vi "Sense.vi"(0 "Enum":enum16{"Running", "Impact", "Spinning", "Clear"}(ring)) -> ()   [LabVIEW 2010]
uses:
  Streaming Data.ctl
  Main Global.vi
panel:
  out "Streaming Data":T1
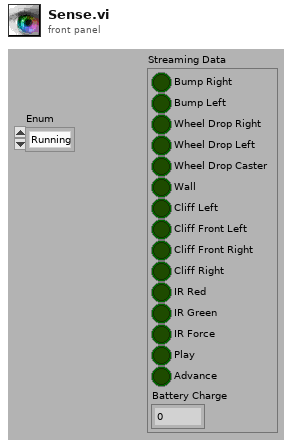
[diagram p1: front panel]
types:
  T1 = typedef "Streaming Data.ctl" = cluster{"Bump Right":bool, "Bump Left":bool, "Wheel Drop Right":bool, "Wheel Drop Left":bool, "Wheel Drop Caster":bool, "Wall":bool, "Cliff Left":bool, "Cliff Front Left":bool, "Cliff Front Right":bool, "Cliff Right":bool, "IR Red":bool, "IR Green":bool, "IR Force":bool, "Play":bool, "Advance":bool, "Battery Charge":i16}
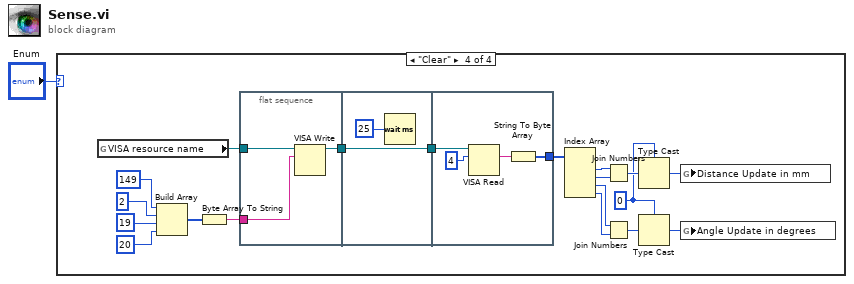
[diagram p0: block diagram]
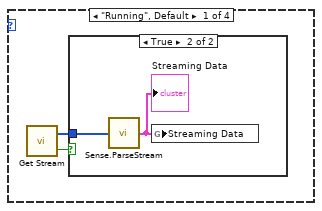
[diagram p2: hidden frame]
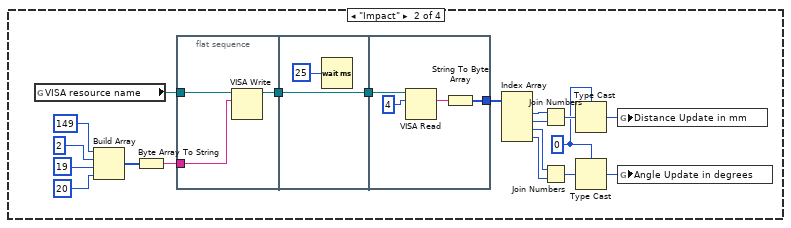
[diagram p4: hidden frame]
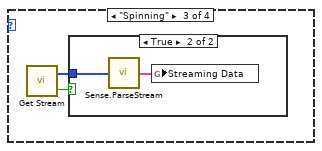
[diagram p5: hidden frame]
diagram:
  n1 = case shown="\"Clear\"" "Enum" {
    frame "Running", Default {
      n2 = call "Get Stream.vi"() -> ("Good Data"=w2:bool, "UART Stream 2"=w3:u8[])  [unwired: 2 in]
      n3 = case shown="True" w2 {
        tunnel: w3 -> [_ w4]
        frame False {
        }
        frame True {
          n4 = call "Sense.ParseStream.vi"("UART Stream"=w4) -> ("Streaming Data"=w5:T1)
          "Streaming Data" <- w5
          n5 = global write "Main Global.vi" "Streaming Data"(w5) -> ()
        }
      }
    }
    frame "Impact" {
      w8 = i16 0
      n6 = global read "Main Global.vi" "VISA resource name"() -> (w24:refnum<visa-resource-name>)
      n7 = Build Array(u8 149, u8 2 ("element"), u8 19, u8 20) -> (w22:u8[])
      n8 = Byte Array To String(unsigned byte array=w22) -> (string=w21:string)
      n9 = flat-sequence {
        tunnel: w24 -> [w27]
        tunnel: w21 -> [w26]
        tunnel: [w25] -> w19
        tunnel: [w28] -> w20
        tunnel: w19 -> [w28]
        tunnel: w20 -> [w33]
        tunnel: [w30] -> w18
        frame #0 {
          n10 = VISA Write(VISA resource name=w27, write buffer=w26) -> (VISA resource name out=w25:refnum<visa-resource-name>)  [unwired: 1 in, 2 out]
        }
        frame #1 {
          n11 = Wait (ms)(milliseconds to wait=u32 25) -> ()  [unwired: 1 out]
        }
        frame #2 {
          n12 = VISA Read(VISA resource name=w33, byte count=u32 4) -> (read buffer=w31:string)  [unwired: 1 in, 3 out]
          n13 = String To Byte Array(string=w31) -> (unsigned byte array=w30:u8[])
        }
      }
      n14 = Index Array(array=w18) -> (element #1=w17:u8, element #2=w16:u8, element #3=w11:u8, element #4=w10:u8)  [unwired: 4 in]
      n15 = Join Numbers(hi=w17, lo=w16) -> ((hi.lo)=w15:u16)
      n16 = Join Numbers(hi=w11, lo=w10) -> ((hi.lo)=w7:u16)
      n17 = Type Cast(type=w8, x=w15) -> (*(type *) &x=w9:i16)
      n18 = Type Cast(type=w8, x=w7) -> (*(type *) &x=w6:i16)
      n19 = global write "Main Global.vi" "Distance Update in mm"(w9) -> ()
      n20 = global write "Main Global.vi" "Angle Update in degrees"(w6) -> ()
    }
    frame "Spinning" {
      n21 = call "Get Stream.vi"() -> ("Good Data"=w35:bool, "UART Stream 2"=w34:u8[])  [unwired: 2 in]
      n22 = case shown="True" w35 {
        tunnel: w34 -> [_ w36]
        frame False {
        }
        frame True {
          n23 = call "Sense.ParseStream.vi"("UART Stream"=w36) -> ("Streaming Data"=w37:T1)
          n24 = global write "Main Global.vi" "Streaming Data"(w37) -> ()
        }
      }
    }
    frame "Clear" {
      w40 = i16 0
      n25 = global read "Main Global.vi" "VISA resource name"() -> (w54:refnum<visa-resource-name>)
      n26 = Build Array(u8 149, u8 2 ("element"), u8 19, u8 20) -> (w52:u8[])
      n27 = Byte Array To String(unsigned byte array=w52) -> (string=w51:string)
      n28 = flat-sequence {
        tunnel: w54 -> [w59]
        tunnel: w51 -> [w58]
        tunnel: [w57] -> w56
        tunnel: [w60] -> w55
        tunnel: w56 -> [w60]
        tunnel: w55 -> [w65]
        tunnel: [w62] -> w50
        frame #0 {
          n29 = VISA Write(VISA resource name=w59, write buffer=w58) -> (VISA resource name out=w57:refnum<visa-resource-name>)  [unwired: 1 in, 2 out]
        }
        frame #1 {
          n30 = Wait (ms)(milliseconds to wait=u32 25) -> ()  [unwired: 1 out]
        }
        frame #2 {
          n31 = VISA Read(VISA resource name=w65, byte count=u32 4) -> (read buffer=w63:string)  [unwired: 1 in, 3 out]
          n32 = String To Byte Array(string=w63) -> (unsigned byte array=w62:u8[])
        }
      }
      n33 = Index Array(array=w50) -> (element #1=w49:u8, element #2=w48:u8, element #3=w43:u8, element #4=w42:u8)  [unwired: 4 in]
      n34 = Join Numbers(hi=w49, lo=w48) -> ((hi.lo)=w47:u16)
      n35 = Join Numbers(hi=w43, lo=w42) -> ((hi.lo)=w39:u16)
      n36 = Type Cast(type=w40, x=w47) -> (*(type *) &x=w41:i16)
      n37 = Type Cast(type=w40, x=w39) -> (*(type *) &x=w38:i16)
      n38 = global write "Main Global.vi" "Distance Update in mm"(w41) -> ()
      n39 = global write "Main Global.vi" "Angle Update in degrees"(w38) -> ()
    }
  }
